vi "__uintSubtract.vi"(7 "Difference (false)":bool, 8 "Base (decimal)":T1=10 items=["Binary"=2, "Octal"=8, "Decimal"=10, "Hexadecimal"=16, "Hexatrigesimal"=36, "ASCII"=64], 10 "Uint2 in":u8[](array[numeric])=[0], 11 "Uint1 in":u8[](array[numeric])=[0]) -> (0 "Timing substraction":u32, 3 "Uint1 - Uint2":u8[](array[numeric]))   [LabVIEW 2011, in "UintClass.lvclass"]
uses:
  UintClass.lvclass
  enumBase.ctl
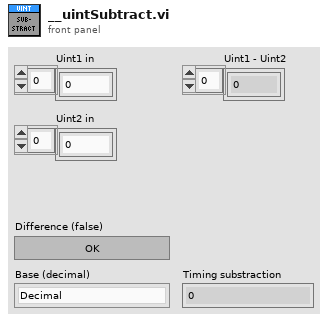
[diagram p1: front panel]
types:
  T1 = typedef "UintClass.lvclass/enumBase.ctl" = u16
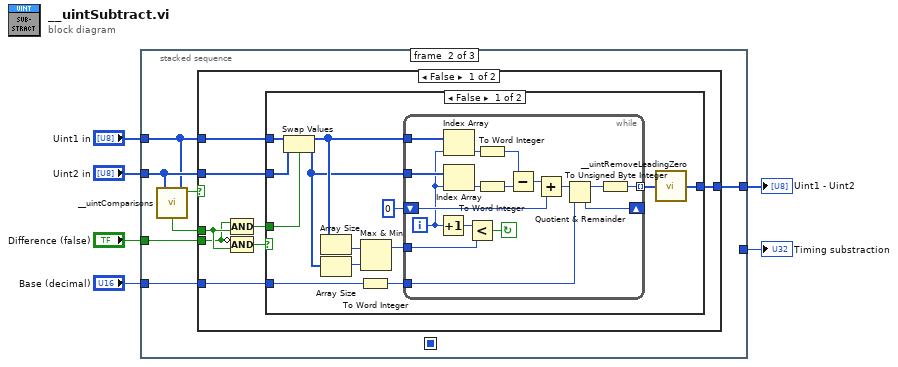
[diagram p0: block diagram]
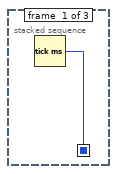
[diagram p2: hidden frame]
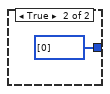
[diagram p3: hidden frame]
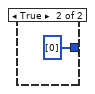
[diagram p4: hidden frame]
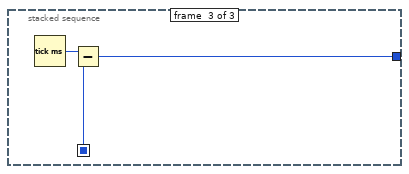
[diagram p5: hidden frame]
diagram:
  n1 = stacked-sequence {
    seq-local: [w7 _ _] -> [_ _ w56]
    tunnel: "Uint1 in" -> [_ w11 _]
    tunnel: "Uint2 in" -> [_ w12 _]
    tunnel: [_ w14 _] -> w6
    tunnel: "Difference (false)" -> [_ w10 _]
    tunnel: "Base (decimal)" -> [_ w9 _]
    tunnel: [_ _ w55] -> w1
    frame #0 {
      n2 = Tick Count (ms)() -> (millisecond timer value=w7:u32)
    }
    frame #1 {
      n3 = call "__uintComparisons.vi"("Uint2 in"=w12, "Uint1 in"=w11) -> ("Uint1 = Uint2"=w8:bool, "Uint1 < Uint2"=w13:bool)  [unwired: 3 in, 5 out]
      n4 = case shown="False" w8 {
        tunnel: [w22 u8[] [0] ("Int out")] -> w14
        tunnel: w13 -> [w21 _]
        tunnel: w12 -> [w20 _]
        tunnel: w11 -> [w19 _]
        tunnel: w10 -> [w18 _]
        tunnel: w9 -> [w17 _]
        frame False {
          n5 = Compound Arithmetic op=AND(w18, w21) -> (w15:bool)
          n6 = Compound Arithmetic op=AND(invert w18, w21) -> (w16:bool)
          n7 = case shown="False" w16 {
            tunnel: [w30 u8[] [0] ("Int out")] -> w22
            tunnel: w20 -> [w26 _]
            tunnel: w19 -> [w27 _]
            tunnel: w17 -> [w29 _]
            tunnel: w15 -> [w23 _]
            frame False {
              n8 = Swap Values(12:w27, 13:w23, 14:w26) -> (1:w25:u8[], 3:w24:u8[])
              n9 = Array Size(array=w25) -> (size(s)=w33:i32)
              n10 = Array Size(array=w24) -> (size(s)=w34:i32)
              n11 = To Word Integer(number=w29) -> (16bit integer=w28:i16)
              n12 = Max & Min(x=w33, y=w34) -> (max(x,y)=w32:i32)  [unwired: 1 out]
              n13 = while {
                tunnel: w25 -> [w52]
                tunnel: w24 -> [w51]
                shift-right: [w47] -> _
                shift-left: i16 0 -> [w48]
                tunnel: [w42] -> w31 mode=indexing
                tunnel: w32 -> [w46]
                tunnel: w28 -> [w40]
                i -> [w45]
                stop <- w36 continue-if-true
                n14 = Increment(x=w45) -> (x+1=w44:i32)
                n15 = Index Array(array=w52, index=w45) -> (element=w50:u8)
                n16 = Index Array(array=w51, index=w45) -> (element=w49:u8)
                n17 = Less?(x=w44, y=w46) -> (x < y?=w36:bool)
                n18 = To Word Integer(number=w50) -> (16bit integer=w39:i16)
                n19 = To Word Integer(number=w49) -> (16bit integer=w38:i16)
                n20 = Subtract(x=w39, y=w38) -> (x-y=w37:i16)
                n21 = Add(x=w37, y=w48) -> (x+y=w43:i16)
                n22 = Quotient & Remainder(x=w43, y=w40) -> (x-y*floor(x/y)=w41:i16, floor(x/y)=w47:i16)
                n23 = To Unsigned Byte Integer(number=w41) -> (unsigned 8bit integer=w42:u8)
              }
              n24 = call "__uintRemoveLeadingZero.vi"("Uint in"=w31) -> ("Uint out"=w30:u8[])
            }
            frame True {
            }
          }
        }
        frame True {
        }
      }
    }
    frame #2 {
      n25 = Tick Count (ms)() -> (millisecond timer value=w57:u32)
      n26 = Subtract(x=w57, y=w56) -> (x-y=w55:u32)
    }
  }
  "Uint1 - Uint2" <- w6
  "Timing substraction" <- w1
